vi "GetFilePath.vi"(8 "error in (no error)":errorcluster, 11 "reference in":refnum<class "TDMS_DataHandler.lvclass">) -> (0 "error out":errorcluster, 2 "Filepath":path, 3 "reference out":refnum<class "TDMS_DataHandler.lvclass">)   [LabVIEW 2019, in "TDMS_DataHandler.lvclass"]
doc: "Pull and update TDMS main file path where TDMS files will be stored"
uses:
  TDMS_DataHandler.lvclass
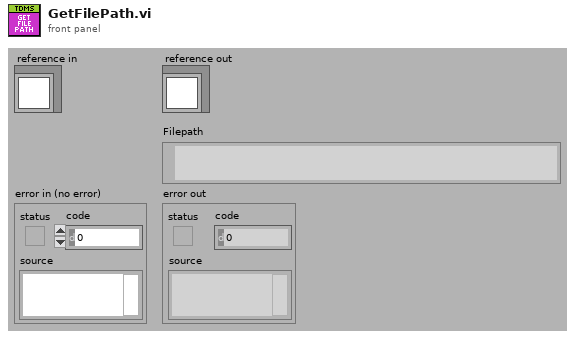
[diagram p1: front panel]
types:
  T1 = typedef "TDMS_DataHandler.lvclass/ObjectAttributesRef.ctl" = refnum<data-value>
  T2 = typedef "TDMS_DataHandler.lvclass/ObjectAttributes.ctl" = cluster{"Directory":path, "FilePath":path, "FileRef":refnum<k34>, "ExperimentName":string, "GroupName":string, "ChannelNames":string[], "Datum":waveform(dbl)[], "Group_Metadata":cluster{"property names":string[], "property values":variant[]}, "Channel_Metadata":cluster{"property names":string[], "property values":variant[]}}
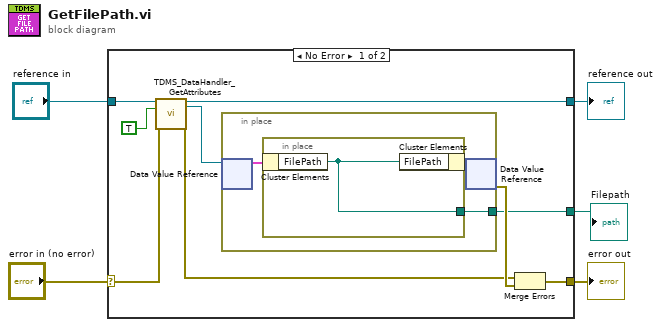
[diagram p0: block diagram]
diagram:
  n1 = case shown="No Error" "error in (no error)" {
    selector: "error in (no error)" -> [w14 w20]
    tunnel: [w8 w20] -> w4
    tunnel: [w13 w19] -> w2
    tunnel: "reference in" -> [w12 w19]
    tunnel: [w6 _] -> w1
    frame No Error {
      n2 = call "TDMS_DataHandler_GetAttributes.vi"("reference in"=w12, "return data? (T)"=TRUE, "error in (no error)"=w14) -> ("reference out"=w13:refnum<class "TDMS_DataHandler.lvclass">, "attributes ref"=w7:T1, "error out"=w9:errorcluster)  [unwired: 13 in, 1 out]
      n3 = in-place {
        in-place-border: [w15] -> w6
        n4 = in-place-dvr #1(w7) -> (w16:T2)  [unwired: 1 out]
        n5 = in-place {
          in-place-border: [w18] -> w15
          n6 = in-place-cluster #2(w16) -> ("FilePath"=w18:path)
          n7 = in-place-cluster #2("FilePath"=w18) -> (w17:T2)
        }
        n8 = in-place-dvr #1(w17) -> (w10:errorcluster)  [unwired: 1 out]
      }
      n9 = Merge Errors(w9, w10) -> (w8:errorcluster)
    }
    frame Error {
    }
  }
  "error out" <- w4
  "reference out" <- w2
  "Filepath" <- w1
